vi "CRAB and II-SLOWCONTR.vi"() -> ()   [LabVIEW 2017]
uses:
  <vilib>/Instr/_visa.llb/VISA Configure Serial Port (Instr).vi
  <instrlib>/BK Precision 913XX/BK Precision 913XX.lvlib
  <vilib>/Analysis/NI_AALBase.lvlib
  <vilib>/Analysis/1siggen.llb/Ramp Pattern by Samples.vi
panel:
  out "Sorted Indexes":i32[](array[numeric])
  in  "Send 4":bool
  out "Message":string
  in  "Reset 4":bool
  out "HV On":bool
  out "Fault":bool
  out "Vmode 4":bool
  out "Imode 4":bool
  out "Voltage Monitor":dbl format="%#.2g"
  out "Current Monitor":dbl format="%#.2g"
  in  "High Voltage":bool
  in  "Voltage Program":dbl min=0.0 max=100.0 step=0.1 format="%#.2g"
  in  "Current Program":dbl min=0.0 max=100.0 step=0.1 format="%#.2g"
  in  "Version 4":bool
  in  "?":bool
  in  "Baud Rate":u16=9600 min=1200 max=19200 step=1200
  in  "Flow Control":u16(ring) items=["None"=0, "XON/XOFF"=1, "RTS/CTS"=2, "DTR/DSR"=4]
  in  "Stop Bits":u16(ring)=10 items=["1.0"=10, "1.5"=15, "2.0"=20]
  in  "Parity":u16(ring) items=["None", "Odd", "Even", "Mark", "Space"]
  in  "Data Bits":u16=8 min=5 max=8 step=1
  in  "VISA resource name":refnum<visa-resource-name>="COM1"
  out "Current Monitor 1":dbl format="%.4g"
  out "Power Monitor 1":dbl format="%.4g"
  out "Voltage Monitor 1":dbl format="%.4g"
  out "Current Monitor 2":dbl format="%.4g"
  out "Power Monitor 2":dbl format="%.4g"
  out "Voltage Monitor 2":dbl format="%.4g"
  out "Current Monitor 3":dbl format="%.4g"
  out "Power Monitor 3":dbl format="%.4g"
  out "Voltage Monitor 3":dbl format="%.4g"
  in  "Voltage Level (0.0 V)":dbl format="%.3g"
  in  "Voltage Level (0.0 V) 2":dbl format="%.3g"
  in  "Voltage Level (0.0 V) 3":dbl format="%.3g"
  in  "Channel (3:3)":u16(ring)=1 items=["1"=1, "2"=2, "3"=3]
  in  "Channel (2:2)":u16(ring)=1 items=["1"=1, "2"=2, "3"=3]
  in  "Channel (1:1)":u16(ring)=1 items=["1"=1, "2"=2, "3"=3]
  in  "Enable OVP":bool=TRUE
  in  "Stop Output":bool
  in  "Voltage Limit":dbl=36.0 min=0.0 max=66.0 step=0.001 format="%.3g"
  in  "Current Limit":dbl min=0.0 max=25.0 step=1.0 format="%.3f"
  in  "VISA resource name":refnum<visa-resource-name>
  in  "Send 3":bool
  out "Message":string
  in  "Reset 3":bool
  out "HV On":bool
  out "Fault":bool
  out "Vmode 3":bool
  out "Imode 3":bool
  out "Voltage Monitor":dbl format="%#.2g"
  out "Current Monitor":dbl format="%#.2g"
  in  "High Voltage":bool
  in  "Voltage Program":dbl min=0.0 max=100.0 step=0.1 format="%#.2g"
  in  "Current Program":dbl min=0.0 max=100.0 step=0.1 format="%#.2g"
  in  "Version 3":bool
  in  "?":bool
  in  "Baud Rate":u16=9600 min=1200 max=19200 step=1200
  in  "Flow Control":u16(ring) items=["None"=0, "XON/XOFF"=1, "RTS/CTS"=2, "DTR/DSR"=4]
  in  "Stop Bits":u16(ring)=10 items=["1.0"=10, "1.5"=15, "2.0"=20]
  in  "Parity":u16(ring) items=["None", "Odd", "Even", "Mark", "Space"]
  in  "Data Bits":u16=8 min=5 max=8 step=1
  in  "VISA resource name":refnum<visa-resource-name>="COM1"
  in  "Send":bool
  in  "Reset":bool
  in  "High Voltage":bool
  in  "Current Program":dbl min=0.0 max=100.0 step=0.1 format="%#.2g"
  in  "Version":bool
  in  "?":bool
  in  "Baud Rate":u16=9600 min=1200 max=19200 step=1200
  in  "Flow Control":u16(ring) items=["None"=0, "XON/XOFF"=1, "RTS/CTS"=2, "DTR/DSR"=4]
  in  "Stop Bits":u16(ring)=10 items=["1.0"=10, "1.5"=15, "2.0"=20]
  in  "Parity":u16(ring) items=["None", "Odd", "Even", "Mark", "Space"]
  in  "Data Bits":u16=8 min=5 max=8 step=1
  in  "VISA resource name":refnum<visa-resource-name>="COM1"
  out "Message":string
  out "HV On":bool
  out "Fault":bool
  out "Vmode":bool
  out "Imode":bool
  out "Voltage Monitor":dbl format="%#.2g"
  out "Current Monitor":dbl format="%#.2g"
  # "LabVIEW Instructions:\n\nAfter all of the VISA resource names have been connected, follow the steps below BEFORE OPERATING CRAB.\n\nFlip HV switch from off to on.\n\nStart program (white arrow on top left). Green \"Voltage Monitor\" light should turn on in the corresponding monitors. Once you send the voltage programs, the red \"HV on\" lights should turn on. Npw, you are ready to operate the CRAB."
  # "I I CONTROLS"
  # "EL + CONTROLS"
  # "FIELD CAGE CONTROLS"
  # "Configuration"
  # "Configuration"
  # "Configuration"
  # "EL+ Instructions:\n\nSet VISA resource name to COM6.\n\nTo start: Set Voltage to 2kV & Current to 0.01 amps\n\nVoltage goes up to 8kV. Slow ramp from 4-8kV in increments of .5kV every 30 seconds. DO NOT EXCEED 8 KV WHEN OPERATING CRAB"
  # "Programs"
  # "Programs"
  # "Programs"
  # "On"
  # "On"
  # "kV"
  # "kV"
  # "[ppsjgsln"
  # "V"
  # "V"
  # "V"
  # "A"
  # "Off"
  # "Off"
  # "A"
  # "EL ++ CONTROLS"
  # "EL++ Instructions:\n\nSet VISA resource name to COM4.\n\nTo start: Set Voltage to 2kV & Current to 0.01 amps\n\nVoltage goes up to 15kV. Slow ramp from 4-15kV in increments of .5kV every 30 seconds. DO NOT EXCEED 18 KV WHEN OPERATING CRAB"
  # "Monitors"
  # "Field Cage Instructions:\n\nSet VISA resource name to COM8.\n\nTo start: Set Voltage to 2kV & Current to 0.01 amps\n\nVoltage goes up to 7kV.\nSlow ramp from 4-7kV in increments of .5kV every 30 seconds. DO NOT EXCEED 8 KV WHEN OPERATING CRAB"
  # "Monitors"
  # "Monitors"
  # "Image Intesnifier Instructions:\n\nSet VISA resource name to USB::0XFFF::0X913....::instr\n\nSet channels accordingly (ie Channel 2 to 2). \n\nSet Voltage limit to 6 and Current limit to 1."
  # "Configuration"
  # "V"
  # "V"
  # "V"
  # "kV"
  # "kV"
  # "V"
  # "V"
  # "V"
  # "A"
  # "A"
  # "Programs"
  # "V"
  # "V"
  # "V"
  # "On"
  # "kV"
  # "Off"
  # "A"
  # "IMAGE INTENSIFIER REGION"
  # "Monitors"
  # "kV"
  # "FIELD CAGE REGION"
  # "A"
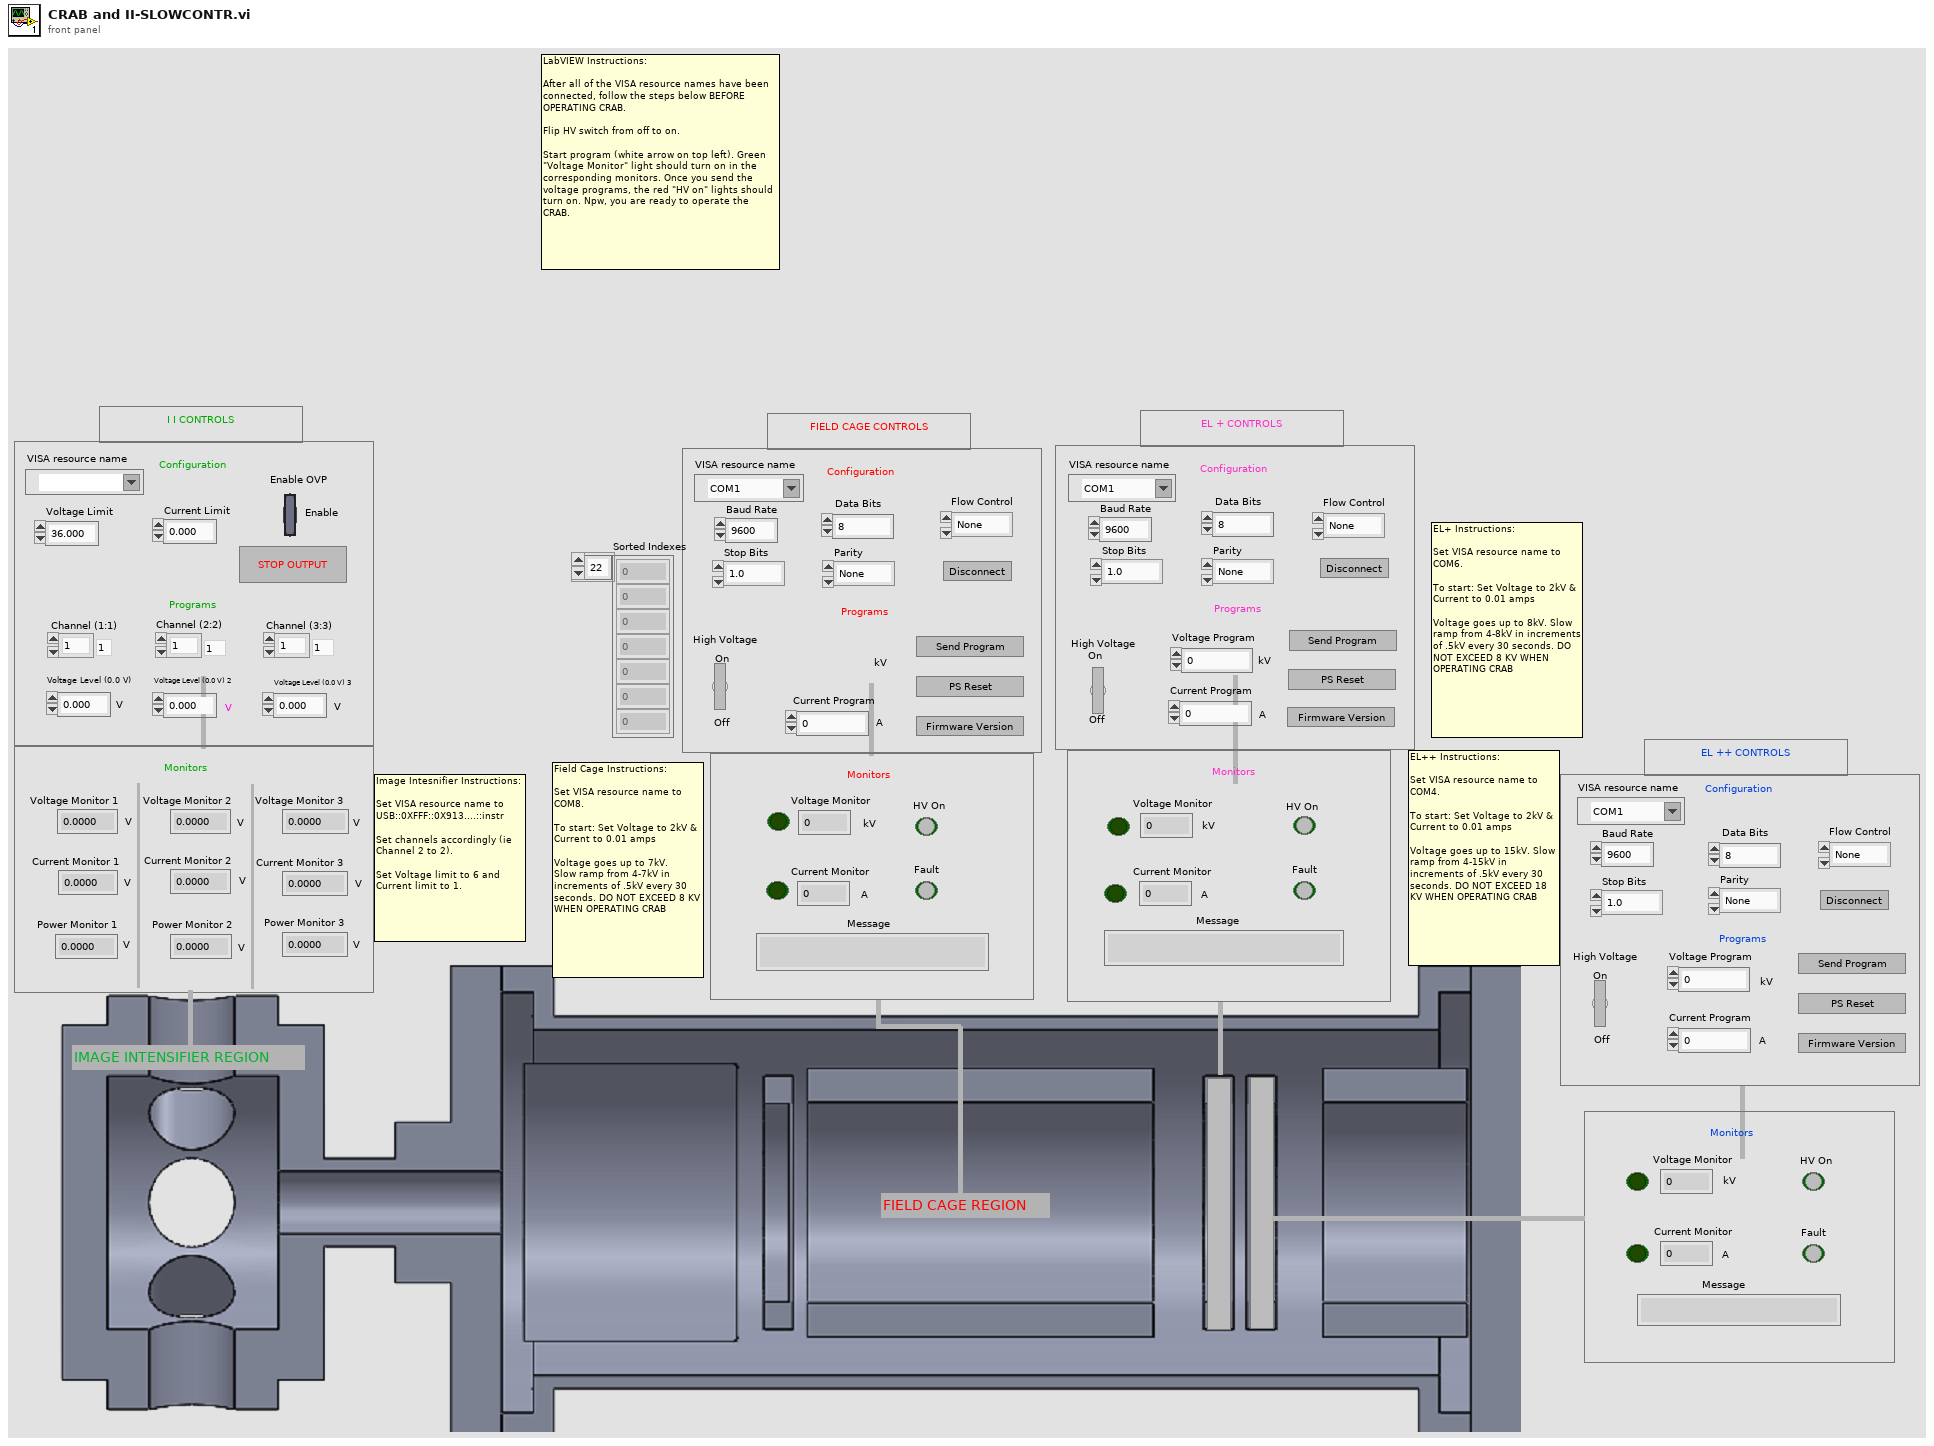
[diagram p1: front panel]
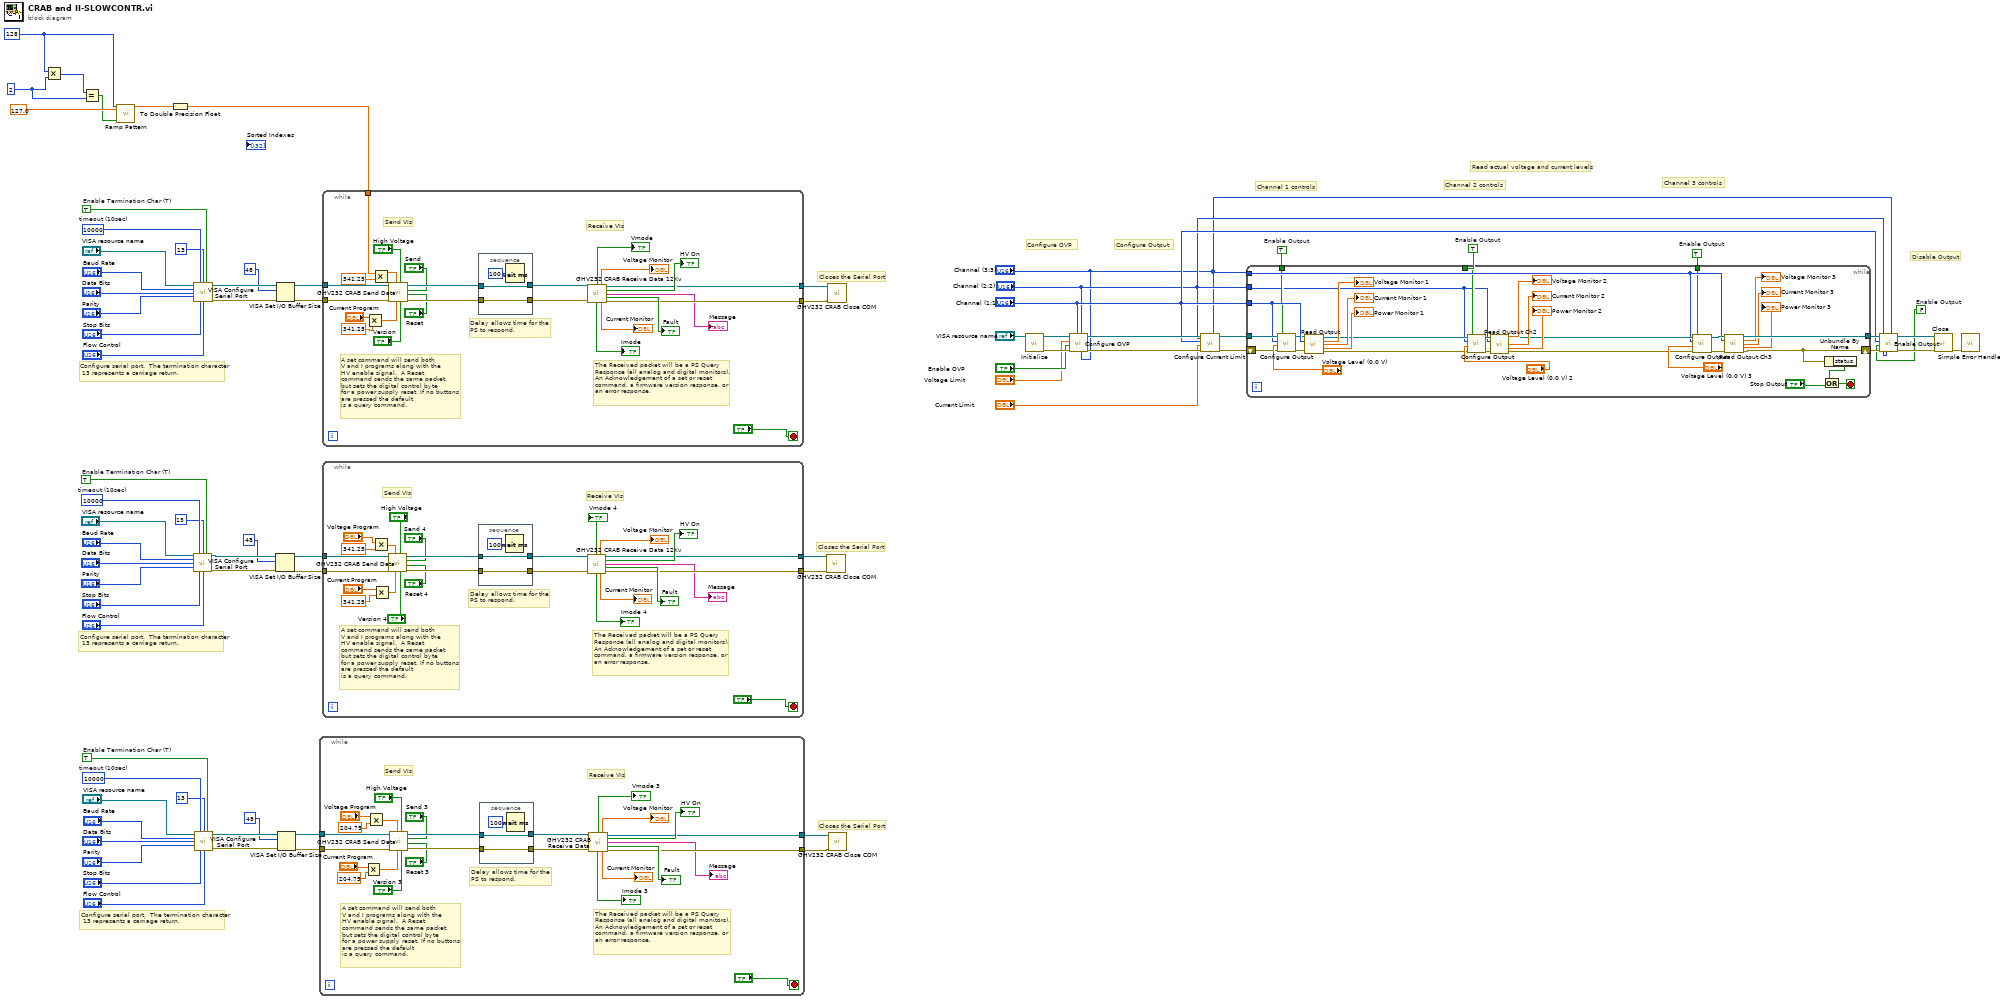
[diagram p0: block diagram]
diagram:
  w3 = 2
  w5 = 128 ("samples")
  w20 = TRUE  # Enable Termination Char (T)
  w21 = u32 10000  # timeout (10sec)
  w26 = TRUE  # Enable Output
  w27 = TRUE  # Enable Output
  w28 = TRUE  # Enable Output
  w30 = FALSE  # Enable Output
  w58 = TRUE  # Enable Termination Char (T)
  w59 = u32 10000  # timeout (10sec)
  w74 = TRUE  # Enable Termination Char (T)
  w75 = u32 10000  # timeout (10sec)
  # "Closes the Serial Port"
  # "Configure serial port.  The termination character\n 13 represents a carriage return."
  # "Channel 3 controls"
  # "Channel 2 controls"
  # "Channel 1 controls"
  # "Disable Output"
  # "Read actual voltage and current levels"
  # "Configure Output"
  # "Configure OVP"
  # "Closes the Serial Port"
  # "Configure serial port.  The termination character\n 13 represents a carriage return."
  # "Closes the Serial Port"
  # "Configure serial port.  The termination character\n 13 represents a carriage return."
  n1 = Multiply(x=w5, y=w3) -> (x*y=w4:i32)
  n2 = Equal?(x=w4, y=w3) -> (x = y?=w6:bool)
  n3 = call-poly <vilib>:"Ramp Pattern.vi"("exclude end?"=w6, "end"=127.0, "samples"=w5) -> ("Ramp Pattern"=w2:dbl[])  [unwired: 7 in, 1 out]
  n4 = To Double Precision Float(number=w2) -> (double precision float=w1:dbl[])
  n5 = call-poly "VISA Configure Serial Port"("VISA resource name"="VISA resource name", "timeout (10sec)"=w21, "termination char\n(0xA = '\\n' = LF)"=13, "Enable Termination\nChar (T)"=w20, "baud rate (9600)"="Baud Rate", "data bits (8)"="Data Bits", "parity (0:none)"="Parity", "stop bits (10: 1 bit)"="Stop Bits", "flow control (0:none)"="Flow Control") -> ("VISA resource name out"=w10:refnum<visa-resource-name>, "error out"=w9:errorcluster)  [unwired: 5 in]
  n6 = call-poly "VISA Configure Serial Port"("VISA resource name"="VISA resource name", "timeout (10sec)"=w75, "termination char\n(0xA = '\\n' = LF)"=13, "Enable Termination\nChar (T)"=w74, "baud rate (9600)"="Baud Rate", "data bits (8)"="Data Bits", "parity (0:none)"="Parity", "stop bits (10: 1 bit)"="Stop Bits", "flow control (0:none)"="Flow Control") -> ("VISA resource name out"=w64:refnum<visa-resource-name>, "error out"=w63:errorcluster)  [unwired: 5 in]
  n7 = call-poly "VISA Configure Serial Port"("VISA resource name"="VISA resource name", "timeout (10sec)"=w59, "termination char\n(0xA = '\\n' = LF)"=13, "Enable Termination\nChar (T)"=w58, "baud rate (9600)"="Baud Rate", "data bits (8)"="Data Bits", "parity (0:none)"="Parity", "stop bits (10: 1 bit)"="Stop Bits", "flow control (0:none)"="Flow Control") -> ("VISA resource name out"=w48:refnum<visa-resource-name>, "error out"=w47:errorcluster)  [unwired: 5 in]
  n8 = VISA Set I/O Buffer Size(VISA resource name=w10, mask (16)=48, error in (no error)=w9) -> (VISA resource name out=w11:refnum<visa-resource-name>, error out=w12:errorcluster)  [unwired: 1 in]
  n9 = VISA Set I/O Buffer Size(VISA resource name=w64, mask (16)=48, error in (no error)=w63) -> (VISA resource name out=w65:refnum<visa-resource-name>, error out=w66:errorcluster)  [unwired: 1 in]
  n10 = VISA Set I/O Buffer Size(VISA resource name=w48, mask (16)=48, error in (no error)=w47) -> (VISA resource name out=w49:refnum<visa-resource-name>, error out=w50:errorcluster)  [unwired: 1 in]
  n11 = while {
    tunnel: w50 -> [w101]
    tunnel: w49 -> [w100]
    tunnel: [w90] -> w52
    tunnel: [w86] -> w51
    stop <- "?" stop-if-true
    # "The Received packet will be a PS Query\nResponse (all analog and digital monitors),\nAn Acknowledgement of a set or reset\ncommand, a firmware version response, or\nan error response."
    # "Delay allows time for the \nPS to respond."
    # "A set command will send both\nV and I programs along with the\nHV enable signal.  A Reset \ncommand sends the same packet,\nbut sets the digital control byte\nfor a power supply reset. If no buttons are pressed the default\nis a query command."
    # "Receive VIs"
    # "Send VIs"
    n12 = Multiply(x="Current Program", y=204.75) -> (x*y=w78:dbl)
    n13 = Multiply(x="Voltage Program", y=204.75) -> (x*y=w81:dbl)
    n14 = call "GHV232 CRAB Send Data.vi"("Reset"="Reset 3", "Send"="Send 3", "Version"="Version 3", "HV Enable"="High Voltage", "Current Program"=w78, "Voltage Program"=w81, "error in (no error)"=w101, "VISA resource name"=w100) -> ("error out"=w103:errorcluster, "VISA resource name 2"=w102:refnum<visa-resource-name>)  [unwired: 2 in]
    n15 = stacked-sequence {
      tunnel: [w106] -> w95
      tunnel: w102 -> [w106]
      tunnel: w103 -> [w105]
      tunnel: [w105] -> w94
      frame #0 {
        n16 = Wait (ms)(milliseconds to wait=100) -> ()  [unwired: 1 out]
      }
    }
    n17 = call "GHV232 CRAB Receive Data.vi"("VISA resource name"=w95, "error in (no error)"=w94) -> ("V"=→"Vmode 3":bool, "Vmon"=→"Voltage Monitor":dbl, "VISA resource name 2"=w90:refnum<visa-resource-name>, "HV on"=→"HV On":bool, "Message"=→"Message":string, "Fault"=→"Fault":bool, "I"=→"Imode 3":bool, "Imon"=→"Current Monitor":dbl, "error out"=w86:errorcluster)  [unwired: 5 in]
  }
  n18 = while {
    tunnel: w12 -> [w130]
    tunnel: w11 -> [w129]
    tunnel: [w120] -> w14
    tunnel: [w116] -> w13
    stop <- "?" stop-if-true
    # "The Received packet will be a PS Query\nResponse (all analog and digital monitors),\nAn Acknowledgement of a set or reset\ncommand, a firmware version response, or\nan error response."
    # "Delay allows time for the \nPS to respond."
    # "A set command will send both\nV and I programs along with the\nHV enable signal.  A Reset \ncommand sends the same packet,\nbut sets the digital control byte\nfor a power supply reset. If no buttons are pressed the default\nis a query command."
    # "Receive VIs"
    # "Send VIs"
    n19 = Multiply(x="Voltage Program", y=341.25) -> (x*y=w113:dbl)
    n20 = Multiply(x="Current Program", y=341.25) -> (x*y=w110:dbl)
    n21 = call "GHV232 CRAB Send Data.vi"("Reset"="Reset 4", "Send"="Send 4", "Version"="Version 4", "HV Enable"="High Voltage", "Current Program"=w110, "Voltage Program"=w113, "error in (no error)"=w130, "VISA resource name"=w129) -> ("error out"=w132:errorcluster, "VISA resource name 2"=w131:refnum<visa-resource-name>)  [unwired: 2 in]
    n22 = stacked-sequence {
      tunnel: [w135] -> w124
      tunnel: w131 -> [w135]
      tunnel: w132 -> [w134]
      tunnel: [w134] -> w123
      frame #0 {
        n23 = Wait (ms)(milliseconds to wait=100) -> ()  [unwired: 1 out]
      }
    }
    n24 = call "GHV232 CRAB Receive Data 12Kv.vi"("VISA resource name"=w124, "error in (no error)"=w123) -> ("V"=→"Vmode 4":bool, "Vmon"=→"Voltage Monitor":dbl, "VISA resource name 2"=w120:refnum<visa-resource-name>, "HV on"=→"HV On":bool, "Message"=→"Message":string, "Fault"=→"Fault":bool, "I"=→"Imode 4":bool, "Imon"=→"Current Monitor":dbl, "error out"=w116:errorcluster)  [unwired: 5 in]
  }
  n25 = while {
    tunnel: w66 -> [w159]
    tunnel: w65 -> [w158]
    tunnel: [w148] -> w68
    tunnel: [w144] -> w67
    tunnel: w1 -> [w137]
    stop <- "?" stop-if-true
    # "The Received packet will be a PS Query\nResponse (all analog and digital monitors),\nAn Acknowledgement of a set or reset\ncommand, a firmware version response, or\nan error response."
    # "Delay allows time for the \nPS to respond."
    # "A set command will send both\nV and I programs along with the\nHV enable signal.  A Reset \ncommand sends the same packet,\nbut sets the digital control byte\nfor a power supply reset. If no buttons are pressed the default\nis a query command."
    # "Receive VIs"
    # "Send VIs"
    n26 = Multiply(x="Current Program", y=341.25) -> (x*y=w138:dbl)
    n27 = Multiply(x=w137, y=341.25) -> (x*y=w136:dbl[])
    n28 = call "GHV232 CRAB Send Data.vi"("Reset"="Reset", "Send"="Send", "Version"="Version", "HV Enable"="High Voltage", "Current Program"=w138, "Voltage Program"=w136, "error in (no error)"=w159, "VISA resource name"=w158) -> ("error out"=w161:errorcluster, "VISA resource name 2"=w160:refnum<visa-resource-name>)  [unwired: 2 in]
    n29 = stacked-sequence {
      tunnel: [w164] -> w153
      tunnel: w160 -> [w164]
      tunnel: w161 -> [w163]
      tunnel: [w163] -> w152
      frame #0 {
        n30 = Wait (ms)(milliseconds to wait=100) -> ()  [unwired: 1 out]
      }
    }
    n31 = call "GHV232 CRAB Receive Data 12Kv.vi"("VISA resource name"=w153, "error in (no error)"=w152) -> ("V"=→"Vmode":bool, "Vmon"=→"Voltage Monitor":dbl, "VISA resource name 2"=w148:refnum<visa-resource-name>, "HV on"=→"HV On":bool, "Message"=→"Message":string, "Fault"=→"Fault":bool, "I"=→"Imode":bool, "Imon"=→"Current Monitor":dbl, "error out"=w144:errorcluster)  [unwired: 5 in]
  }
  n32 = call "GHV232 CRAB Close COM.vi"("error in (no error)"=w13, "VISA resource name"=w14) -> ()  [unwired: 9 in, 1 out]
  n33 = call "GHV232 CRAB Close COM.vi"("error in (no error)"=w67, "VISA resource name"=w68) -> ()  [unwired: 9 in, 1 out]
  n34 = call "GHV232 CRAB Close COM.vi"("error in (no error)"=w51, "VISA resource name"=w52) -> ()  [unwired: 9 in, 1 out]
  n35 = call <instrlib>:"Initialize.vi"("VISA resource name"="VISA resource name") -> ("error out"=w43:errorcluster, "VISA resource name out"=w42:refnum<visa-resource-name>)  [unwired: 9 in]
  n36 = call <instrlib>:"Configure OVP.vi"("Channel (3:3)"="Channel (3:3)", "Channel (2:2)"="Channel (2:2)", "Channel (1:1)"="Channel (1:1)", "error in (no error)"=w43, "Enable OVP (T: Enable)"="Enable OVP", "Voltage Limit (36.000 V)"="Voltage Limit", "VISA resource name"=w42) -> ("error out"=w40:errorcluster, "VISA resource name out"=w41:refnum<visa-resource-name>)  [unwired: 3 in]
  n37 = call <instrlib>:"Configure Current Limit.vi"("Channel (3:3)"="Channel (3:3)", "Channel (2:2)"="Channel (2:2)", "error in (no error)"=w40, "Current Limit (0.0 A)"="Current Limit", "Channel (1:1)"="Channel (1:1)", "VISA resource name"=w41) -> ("error out"=w36:errorcluster, "VISA resource name out"=w35:refnum<visa-resource-name>)  [unwired: 4 in]
  n38 = while {
    tunnel: w35 -> [w193]
    tunnel: [w190] -> w39
    shift-right: [w166] -> w34
    shift-left: w36 -> [w172]
    tunnel: "Channel (1:1)" -> [w192]
    tunnel: "Channel (2:2)" -> [w165]
    tunnel: "Channel (3:3)" -> [w179]
    tunnel: w28 -> [w178]
    tunnel: w27 -> [w174]
    tunnel: w26 -> [w177]
    stop <- w199 stop-if-true
    n39 = call <instrlib>:"Configure Output.vi"("Enable Channel Output (F: False)"=w178, "error in (no error)"=w172, "Voltage Level (0.0 V)"="Voltage Level (0.0 V)", "Channel (1:1)"=w192, "VISA resource name"=w193) -> ("error out"=w171:errorcluster, "VISA resource name out"=w182:refnum<visa-resource-name>)  [unwired: 5 in]
    n40 = call <instrlib>:"Read Output.vi"("VISA resource name"=w182, "Channel (1:Channel 1)"=w192, "error in (no error)"=w171) -> ("VISA resource name out"=w175:refnum<visa-resource-name>, "Actual Voltage Level (V)"=→"Voltage Monitor 1":dbl, "Actual Current Level (A)"=→"Current Monitor 1":dbl, "Actual Power Level (W)"=→"Power Monitor 1":dbl, "error out"=w170:errorcluster)  [unwired: 8 in]
    n41 = call <instrlib>:"Configure Output.vi"("Enable Channel Output (F: False)"=w174, "error in (no error)"=w170, "Voltage Level (0.0 V)"="Voltage Level (0.0 V) 2", "Channel (1:1)"=w165, "VISA resource name"=w175) -> ("error out"=w169:errorcluster, "VISA resource name out"=w176:refnum<visa-resource-name>)  [unwired: 5 in]
    n42 = call <instrlib>:"Read Output Ch2.vi"("VISA resource name"=w176, "Channel (1:Channel 1)"=w165, "error in (no error)"=w169) -> ("VISA resource name out"=w181:refnum<visa-resource-name>, "Actual Voltage Level (V)"=→"Voltage Monitor 2":dbl, "Actual Current Level (A)"=→"Current Monitor 2":dbl, "Actual Power Level (W)"=→"Power Monitor 2":dbl, "error out"=w168:errorcluster)  [unwired: 8 in]
    n43 = call <instrlib>:"Configure Output.vi"("Enable Channel Output (F: False)"=w177, "error in (no error)"=w168, "Voltage Level (0.0 V)"="Voltage Level (0.0 V) 3", "Channel (1:1)"=w179, "VISA resource name"=w181) -> ("error out"=w167:errorcluster, "VISA resource name out"=w180:refnum<visa-resource-name>)  [unwired: 5 in]
    n44 = call <instrlib>:"Read Output Ch3.vi"("VISA resource name"=w180, "Channel (1:Channel 1)"=w179, "error in (no error)"=w167) -> ("VISA resource name out"=w190:refnum<visa-resource-name>, "Actual Voltage Level (V)"=→"Voltage Monitor 3":dbl, "Actual Current Level (A)"=→"Current Monitor 3":dbl, "Actual Power Level (W)"=→"Power Monitor 3":dbl, "error out"=w166:errorcluster)  [unwired: 8 in]
    n45 = Unbundle By Name(w166) -> ("status"=w197:bool)
    n46 = Or(x=w197, y="Stop Output") -> (x .or. y?=w199:bool)
  }
  n47 = call <instrlib>:"Enable Output.vi"("Channel (3:3)"="Channel (3:3)", "Channel (2:2)"="Channel (2:2)", "error in (no error)"=w34, "Enable Output (F: False)"=w30, "Channel (1:1)"="Channel (1:1)", "VISA resource name"=w39) -> ("error out"=w37:errorcluster, "VISA resource name out"=w38:refnum<visa-resource-name>)  [unwired: 4 in]
  n48 = call <instrlib>:"Close.vi"("error in (no error)"=w37, "VISA resource name"=w38) -> ("error out"=w44:errorcluster)  [unwired: 9 in]
  n49 = call <vilib>:"Simple Error Handler.vi"("error in (no error)"=w44) -> ()  [unwired: 4 in, 5 out]
